vi "Build Read.vi"(4 "Limit":i64, 6 "Where":string, 8 "error in (no error)":errorcluster, 9 "tableName":string, 10 "DynamicParameters in":refnum<class "DynamicParameters.lvclass">, 11 "KDBConnection in":refnum<class "DBC.lvclass">) -> (0 "error out":errorcluster, 2 "Query":string, 3 "KDBConnection out":refnum<class "DBC.lvclass">)   [LabVIEW 2020, in "ORM_DBC_Kdb.lvlib" / "DBC.lvclass"]
uses:
  DBC.lvclass
  C:/Program Files/National Instruments/LabVIEW 2020/vi.lib/Viviota/shared/ORM.lvlibp/ORM/DbConnection/DbConnection.lvclass
  <vilib>/Viviota/shared/ORM.lvlibp/ORM/DynamicParameters/DynamicParameters.lvclass
  <vilib>/Viviota/shared/ORM.lvlibp/ORM/DbConnection/Read ColumnNameEqualsValueFormat.vi
  <vilib>/Viviota/shared/ORM.lvlibp/ORM/DynamicParameters/Read FieldNames.vi
  <vilib>/Viviota/shared/ORM.lvlibp/ORM/DynamicParameters/Read ParameterNames.vi
  <vilib>/Viviota/shared/ORM.lvlibp/ORM/DynamicParameters/Read RequestedFields.vi
  <vilib>/Viviota/shared/ORM.lvlibp/ORM/DynamicParameters/Read AutoKey.vi
  <vilib>/Viviota/shared/ORM.lvlibp/ORM/DynamicParameters/Read ParameterOptions.vi
  <vilib>/regexp/Match Regular Expression.xnode
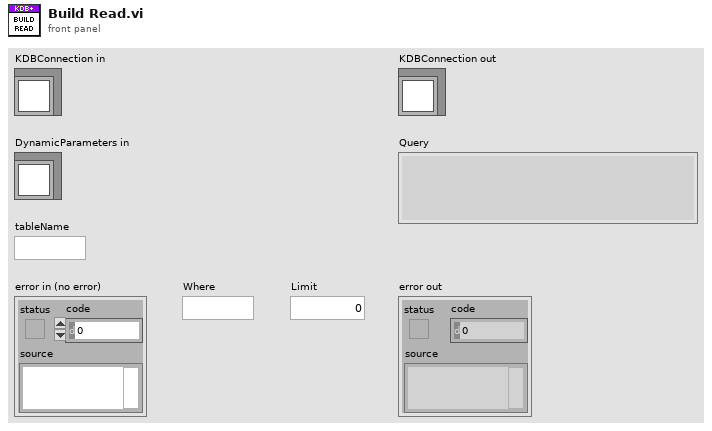
[diagram p1: front panel]
types:
  T1 = cluster{"DbType":i32, "Direction":i32, "Size":i32, "Precision":u8, "Scale":u8}[]
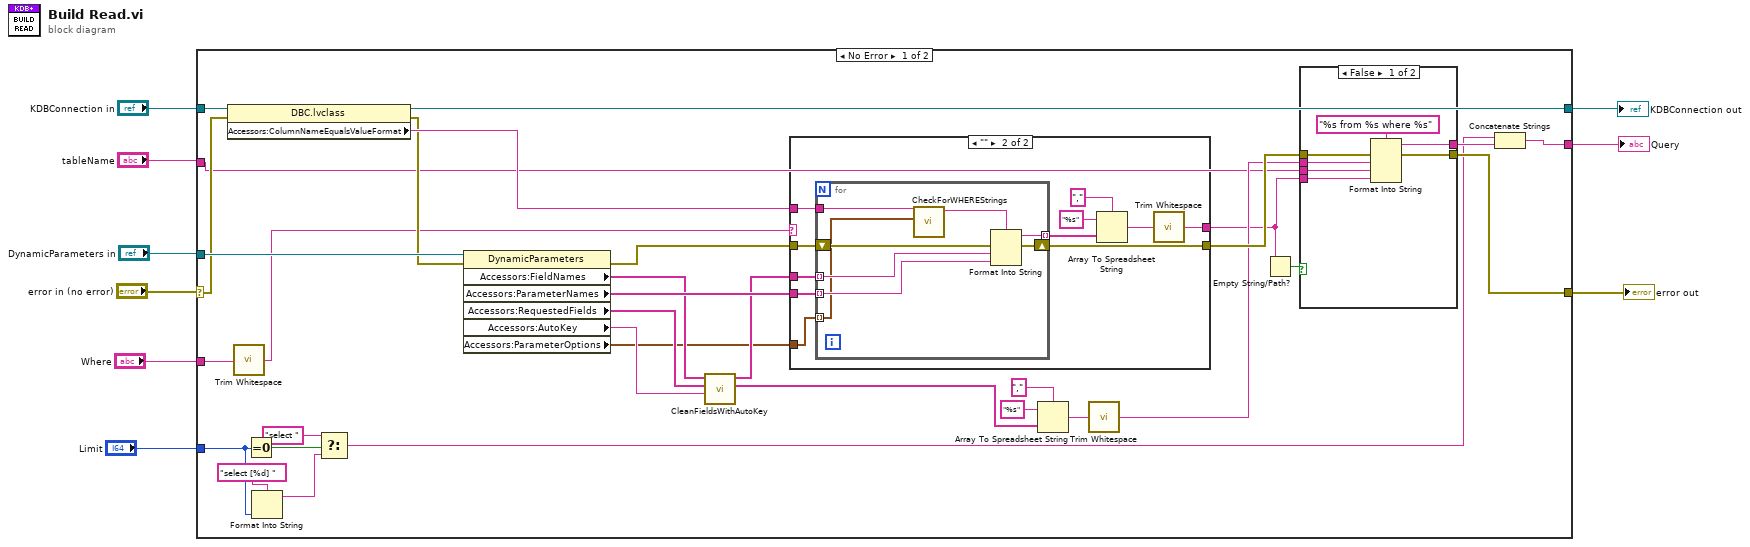
[diagram p0: block diagram]
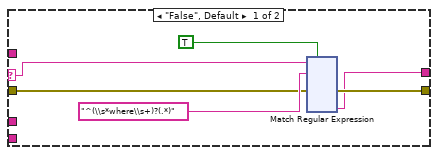
[diagram p2: hidden frame]
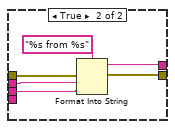
[diagram p3: hidden frame]
diagram:
  n1 = case shown="No Error" "error in (no error)" {
    selector: "error in (no error)" -> [w36 w199]
    tunnel: [w32 w199] -> w4
    tunnel: [w41 w198] -> w8
    tunnel: "KDBConnection in" -> [w42 w198]
    tunnel: "DynamicParameters in" -> [w40 _]
    tunnel: "tableName" -> [w22 _]
    tunnel: [w12 _] -> w3
    tunnel: "Where" -> [w21 _]
    tunnel: "Limit" -> [w17 _]
    frame No Error {
      n2 = property class="DBC.lvclass"(reference=w42, error in=w36) -> (reference out=w41:refnum<class "DBC.lvclass">, error out=w35:errorcluster, "Accessors:ColumnNameEqualsValueFormat"=w38:string)
      n3 = call <vilib>:"Trim Whitespace.vi"("string"=w21) -> ("trimmed string"=w20:string)  [unwired: 1 in]
      n4 = Equal To 0?(x=w17) -> (x = 0?=w15:bool)
      n5 = Format Into String(format string="select [%d] ", w17) -> (resulting string=w14:string)  [unwired: 2 in, 1 out]
      n6 = Select(t="select ", s=w15, f=w14) -> (s? t:f=w11:string)
      n7 = property class="DynamicParameters"(reference=w40, error in=w35) -> (error out=w34:errorcluster, "Accessors:FieldNames"=w31:string[], "Accessors:ParameterNames"=w39:string[], "Accessors:RequestedFields"=w30:string[], "Accessors:AutoKey"=w29:string, "Accessors:ParameterOptions"=w10:T1)  [unwired: 1 out]
      n8 = call "CleanFieldsWithAutoKey.vi"("AutoKey"=w29, "RequestedFields"=w30, "FieldNames"=w31) -> ("RequestedFields_Clean"=w24:string[], "FieldNames_Clean"=w28:string[])  [unwired: 7 in]
      n9 = case shown="\"\"" w20 {
        selector: w20 -> [w43 _]
        tunnel: w39 -> [_ w176]
        tunnel: w38 -> [_ w175]
        tunnel: w34 -> [w46 w170]
        tunnel: [w45 w169] -> w33
        tunnel: w28 -> [_ w168]
        tunnel: [w44 w167] -> w18
        tunnel: w10 -> [_ w166]
        frame "False", Default {
          n10 = xnode "Match Regular Expression"("input string"=w43, "regular expression"="^(\\s*where\\s+)?(.*)", "error in"=w46, "ignore case? (F)"=TRUE) -> ("error out"=w45:errorcluster, "submatch 2"=w44:string)  [unwired: 2 in, 5 out]
        }
        frame "" {
          n11 = for {
            tunnel: w168 -> [w184] mode=indexing
            tunnel: w176 -> [w183] mode=indexing
            tunnel: w175 -> [w178]
            tunnel: [w182] -> w172 mode=indexing
            shift-right: [w180] -> w169
            shift-left: w170 -> [w181]
            tunnel: w166 -> [w179] mode=indexing
            n12 = call "CheckForWHEREStrings.vi"("Options"=w179, "ColumnNameEqualsValueFormat in"=w178) -> ("ColumnNameEqualsValueFormat out"=w177:string)  [unwired: 9 in]
            n13 = Format Into String(format string=w177, error in=w181, w184, w183) -> (resulting string=w182:string, error out=w180:errorcluster)  [unwired: 1 in]
          }
          n14 = Array To Spreadsheet String(delimiter (Tab)=",", array=w172, 3:"%s" ("format string")) -> (spreadsheet string=w174:string)
          n15 = call <vilib>:"Trim Whitespace.vi"("string"=w174) -> ("trimmed string"=w167:string)  [unwired: 1 in]
        }
      }
      n16 = Array To Spreadsheet String(delimiter (Tab)=",", array=w24, 3:"%s" ("format string")) -> (spreadsheet string=w25:string)
      n17 = call <vilib>:"Trim Whitespace.vi"("string"=w25) -> ("trimmed string"=w23:string)  [unwired: 1 in]
      n18 = Empty String/Path?(string/path=w18) -> (empty?=w19:bool)
      n19 = case shown="False" w19 {
        tunnel: [w190 w194] -> w37
        tunnel: w33 -> [w189 w197]
        tunnel: [w188 w196] -> w32
        tunnel: w23 -> [w187 w193]
        tunnel: w18 -> [w186 _]
        tunnel: w22 -> [w185 w192]
        frame False {
          n20 = Format Into String(format string="%s from %s where %s", error in=w189, w187, w185, w186) -> (resulting string=w190:string, error out=w188:errorcluster)  [unwired: 1 in]
        }
        frame True {
          n21 = Format Into String(format string="%s from %s", error in=w197, w193, w192) -> (resulting string=w194:string, error out=w196:errorcluster)  [unwired: 1 in]
        }
      }
      n22 = Concatenate Strings(w11, w37) -> (w12:string)
    }
    frame Error {
    }
  }
  "error out" <- w4
  "KDBConnection out" <- w8
  "Query" <- w3
